vi "FP_Full_Screen_2016.vi"() -> ()   [LabVIEW 2021]
uses:
  <vilib>/Utility/miscctls.llb/LVRectTypeDef.ctl
panel:
  in  "stop":bool
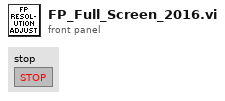
[diagram p1: front panel]
types:
  T1 = typedef "LVRectTypeDef.ctl" = cluster{"Left":i16, "Top":i16, "Right":i16, "Bottom":i16}
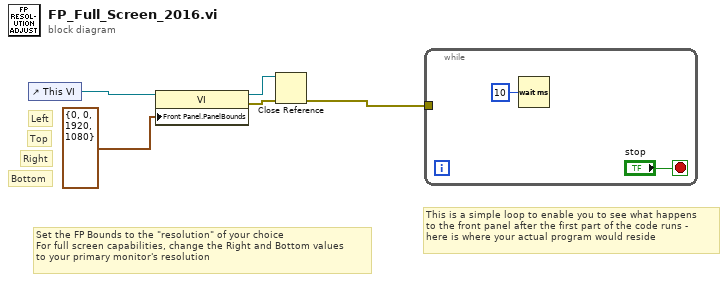
[diagram p0: block diagram]
diagram:
  # "This is a simple loop to enable you to see what happens\nto the front panel after the first part of the code runs - \nhere is where your actual program would reside"
  # "Set the FP Bounds to the \"resolution\" of your choice\nFor full screen capabilities, change the Right and Bottom values\nto your primary monitor's resolution"
  # "Bottom"
  # "Right"
  # "Top"
  # "Left"
  n1 = control-ref of="This VI"() -> (w5:refnum<vi>)
  n2 = property class="VI"(reference=w5, "Front Panel.PanelBounds"=T1 {"Left"=0, "Top"=0, "Right"=1920, "Bottom"=1080} ("Front Panel Window:Panel Bounds")) -> (reference out=w2:refnum<vi>, error out=w3:errorcluster)  [unwired: 1 in]
  n3 = Close Reference(reference=w2, error in (no error)=w3) -> (error out=w1:errorcluster)
  n4 = while {
    tunnel: w1 -> [_]
    stop <- "stop" stop-if-true
    n5 = Wait (ms)(milliseconds to wait=u32 10) -> ()  [unwired: 1 out]
  }
